vi "LHF.DB.Mongo.Client.GetDatabasesName.vi"(0 "LHF.DB.Mongo":refnum<class "LHF.DB.Mongo.lvclass">, 5 "error in (no error)":errorcluster) -> (14 "LHF.DB.Mongo":refnum<class "LHF.DB.Mongo.lvclass">, 15 "Databases":string[](array[string]), 19 "error out":errorcluster)   [LabVIEW 2013, in "LHF.DB.Mongo.lvclass"]
uses:
  LHF.DB.Mongo.lvclass
  LHF.DB.Mongo.lvclass/LHF.DB.Mongo.ctl
  C:/Users/Ricardo/Desktop/Projetos/LabVIEW-MongoDB/src/Driver/MongoDB.Driver.dll
  LabVIEW-MongoDB/src/Driver/MongoDB.Driver.dll
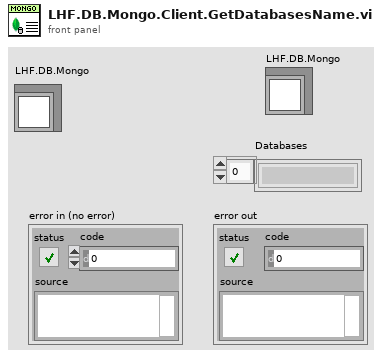
[diagram p1: front panel]
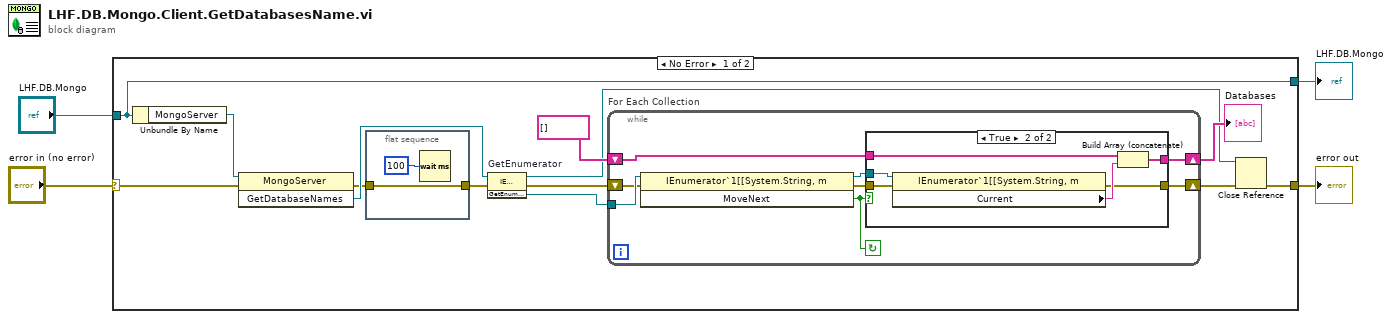
[diagram p0: block diagram]
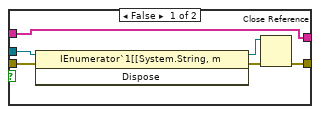
[diagram p2: hidden frame]
diagram:
  n1 = case shown="No Error" "error in (no error)" {
    selector: "error in (no error)" -> [w6 w41]
    tunnel: "LHF.DB.Mongo" -> [w5 w40]
    tunnel: [w7 w41] -> w4
    tunnel: [w5 w40] -> w1
    frame No Error {
      n2 = Unbundle By Name(w5) -> ("MongoServer"=w12:refnum<k24>)
      n3 = invoke class="MongoServer" method="GetDatabaseNames"(reference=w12, error in=w6) -> (error out=w10:errorcluster, "GetDatabaseNames"=w15:refnum<k24>)  [unwired: 1 in, 1 out]
      n4 = flat-sequence {
        tunnel: [w18] -> w11
        tunnel: w10 -> [w18]
        frame #0 {
          n5 = Wait (ms)(milliseconds to wait=u32 100) -> ()  [unwired: 1 out]
        }
      }
      n6 = invoke on="GetEnumerator" class="IEnumerable`1[[System.String, m" method="GetEnumerator"(reference=w15, error in=w11) -> (reference out=w8:refnum<k24>, error out=w16:errorcluster, "GetEnumerator"=w14:refnum<k24>)  [unwired: 1 in]
      n7 = while "For Each Collection" {
        tunnel: w14 -> [w27]
        shift-right: [w22] -> w17
        shift-left: string[] [] -> [w21]
        shift-right: [w20] -> w9
        shift-left: w16 -> [w23]
        stop <- w25 continue-if-true
        n8 = invoke class="IEnumerator`1[[System.String, m" method="MoveNext"(reference=w27, error in=w23) -> (reference out=w26:refnum<k24>, error out=w24:errorcluster, "MoveNext"=w25:bool)  [unwired: 1 in]
        n9 = case shown="True" w25 {
          tunnel: w26 -> [w32 w39]
          tunnel: w24 -> [w29 w38]
          tunnel: [w33 w37] -> w22
          tunnel: w21 -> [w33 w36]
          tunnel: [w28 w34] -> w20
          frame False {
            n10 = invoke class="IEnumerator`1[[System.String, m" method="Dispose"(reference=w32, error in=w29) -> (reference out=w31:refnum<k24>, error out=w30:errorcluster)  [unwired: 1 in, 1 out]
            n11 = Close Reference(reference=w31, error in (no error)=w30) -> (error out=w28:errorcluster)
          }
          frame True {
            n12 = property class="IEnumerator`1[[System.String, m"(reference=w39, error in=w38) -> (error out=w34:errorcluster, "Current"=w35:string)  [unwired: 1 out]
            n13 = Build Array (concatenate)(w36, w35) -> (w37:string[])
          }
        }
      }
      "Databases" <- w17
      n14 = Close Reference(reference=w8, error in (no error)=w9) -> (error out=w7:errorcluster)
    }
    frame Error {
    }
  }
  "error out" <- w4
  "LHF.DB.Mongo" <- w1
